vi "Main Window.vi"() -> ()   [LabVIEW 2014]
uses:
  Temp Sensor Folder/Global Stop TempSensor.vi
  StopForLog.vi
panel:
  in  "בחירה חופשית":bool caption="Blank Button"
  in  "ממסר השהייה למפוח מפנה גזים 0410-26308":bool caption="Blank Button"
  in  "ממסר דימום מנוע 0410-26294":bool caption="Blank Button"
  in  "0410-24534 15A ממסר":bool caption="Blank Button"
  in  "0410-19646 10Ax4 ממסר":bool caption="Blank Button"
  in  "תיבת נתיכים סימן 4 0414-83040":bool caption="Blank Button"
  in  "תיבת מפעיל ריצוף 1469-98836":bool caption="Blank Button"
  in  "תיבת הזנה כיס צריח 0410-23813":bool caption="Blank Button"
  in  "Help Button":bool
  in  "Stop Button":bool
  out "error IO":errorcluster
  in  "error":errorcluster
  # "צב\"ד לממסרים ונתיכים"
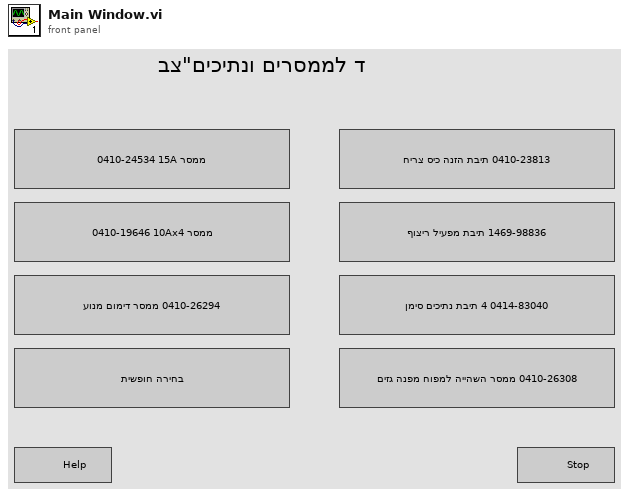
[diagram p1: front panel]
types:
  T1 = enum32{"Invalid", "Standard", "Closed", "Hidden", "Minimized", "Maximized"}
  T2 = enum16{"open", "replace", "create", "open or create", "replace or create", "replace or create with confirmation"}
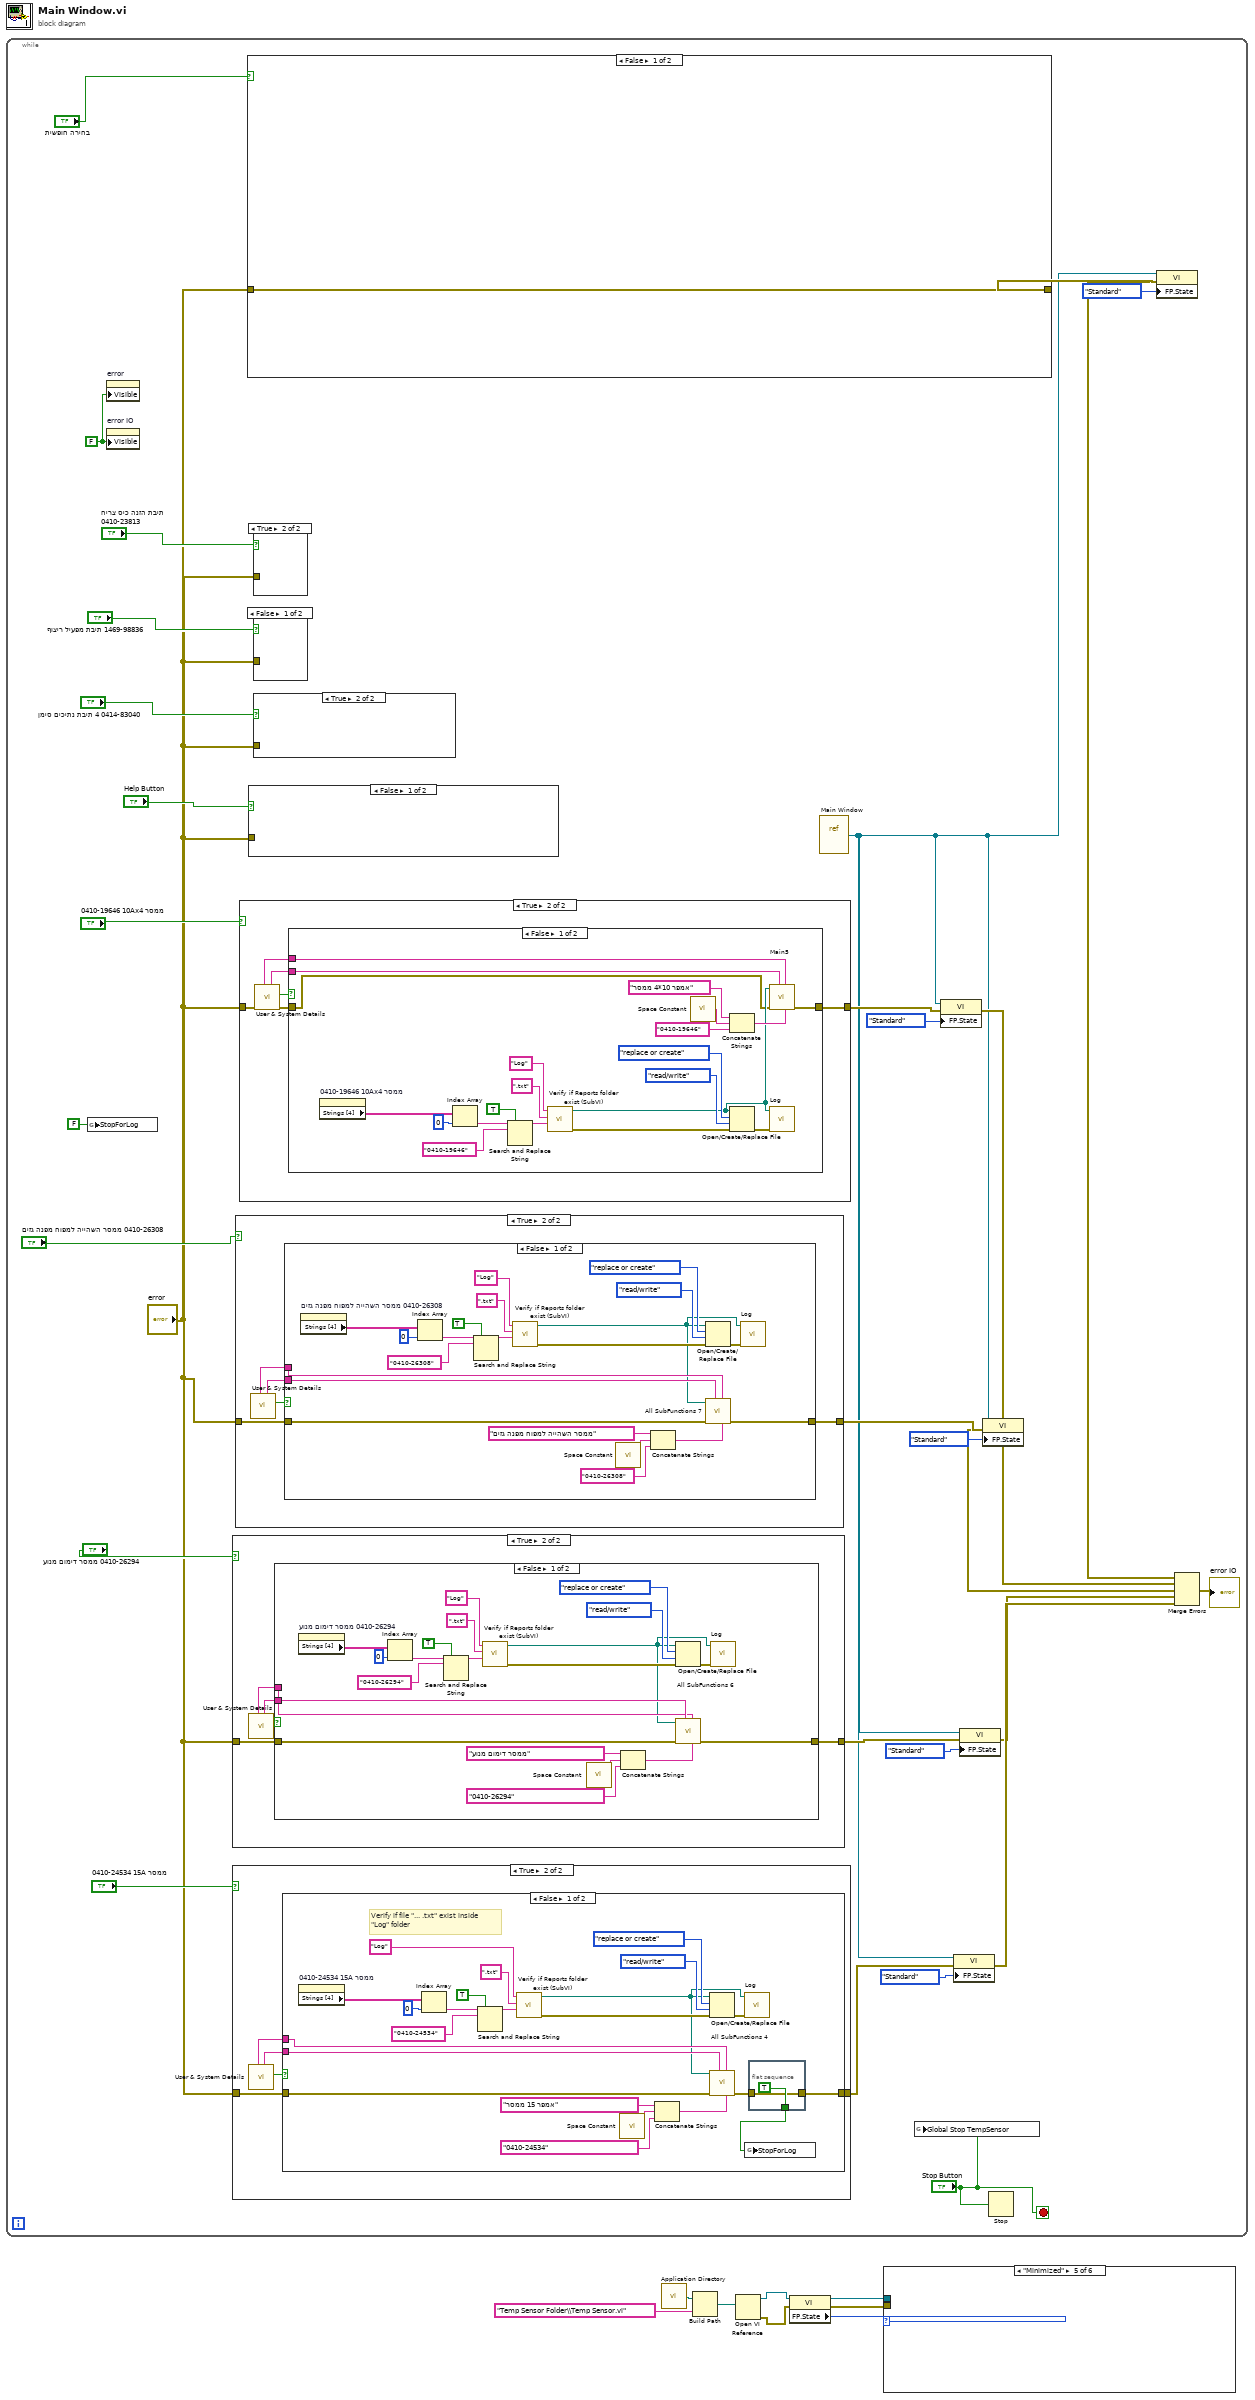
[diagram p0: block diagram]
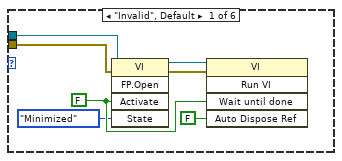
[diagram p2: hidden frame]
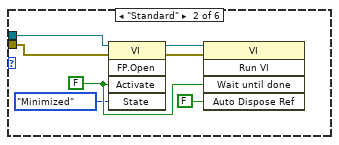
[diagram p3: hidden frame]
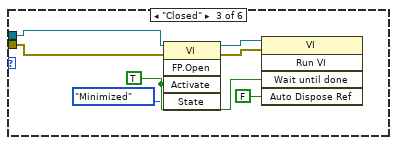
[diagram p4: hidden frame]
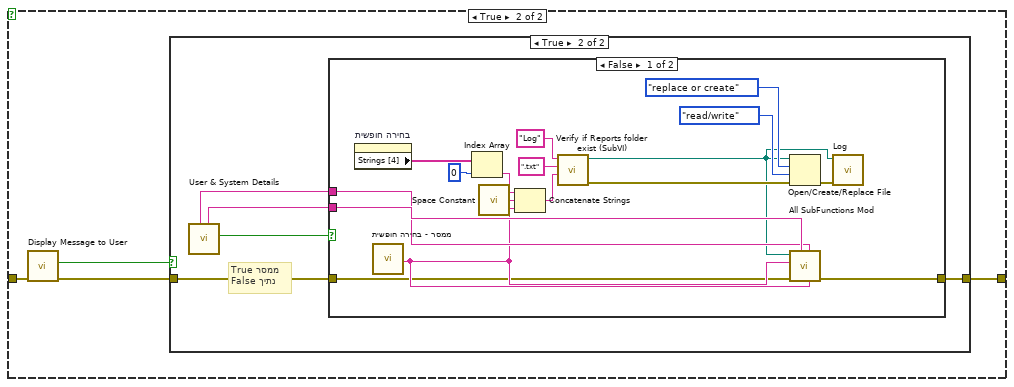
[diagram p7: hidden frame]
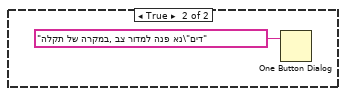
[diagram p10: hidden frame]
diagram:
  n1 = while {
    stop <- "Stop Button" stop-if-true
    w30 = FALSE ("Visible")
    n2 = global write "StopForLog.vi" "StopForLog"(FALSE ("StopForLog")) -> ()
    n3 = property on="error" class="Clust (strict)"("Visible"=w30) -> ()  [unwired: 2 in, 2 out]
    n4 = property on="error IO" class="Clust (strict)"("Visible"=w30) -> ()  [unwired: 2 in, 2 out]
    n5 = case shown="True" "ממסר דימום מנוע 0410-26294" {
      tunnel: "error" -> [w158 w163]
      tunnel: [w158 w162] -> w25
      frame False {
      }
      frame True {
        n6 = call "User & System Details.vi"() -> ("Boolean"=w161:bool, "User Name 2"=w160:string, "מספר סידורי 2"=w159:string)  [unwired: 8 in, 1 out]
        n7 = case shown="False" w161 {
          tunnel: w163 -> [w165 w185]
          tunnel: [w167 w185] -> w162
          tunnel: w160 -> [w169 _]
          tunnel: w159 -> [w168 _]
          frame False {
            n8 = property on="ממסר דימום מנוע 0410-26294" class="Bool"() -> ("Strings [4]"=w176:string[])  [unwired: 2 in, 2 out]
            n9 = Index Array(array=w176, index=0) -> (element=w181:string)
            n10 = Search and Replace String(replace all?=TRUE ("replace all? (F)"), input string=w181, search string="0410-26294") -> (result string=w179:string)  [unwired: 5 in, 3 out]
            n11 = call "Verify if Reports folder exist (SubVI).vi"("שם הממסר"=w179, "File Type"=".txt", "Folder Name"="Log" ("string")) -> ("error out"=w173:errorcluster, "Path"=w164:path)  [unwired: 7 in]
            n12 = call <vilib>:"Space Constant.vi"() -> ("String"=w184:string)
            n13 = Concatenate Strings("ממסר דימום מנוע", w184, "0410-26294") -> (w170:string)
            n14 = Open/Create/Replace File(file path (use dialog)=w164, error in=w173, operation (0:open)=T2."replace or create", access (0:read/write)=enum16{"read/write", "read-only", "write-only"}."read/write") -> (error out=w166:errorcluster)  [unwired: 2 in, 2 out]
            n15 = call "All SubFunctions 6.vi"("מק\"ט המכלל"=w170, "מספר סידורי"=w168, "מפעיל"=w169, "error"=w165, "Path for Log"=w164) -> ("error IO"=w167:errorcluster)  [unwired: 6 in]
            n16 = call "Log.vi"("error in"=w166, "File Path Control"=w164) -> ()  [unwired: 8 in, 2 out]
          }
          frame True {
          }
        }
      }
    }
    n17 = case shown="True" "0410-24534 15A ממסר" {
      tunnel: "error" -> [w69 w70]
      tunnel: [w69 w74] -> w28
      frame False {
      }
      frame True {
        n18 = call "User & System Details.vi"() -> ("Boolean"=w73:bool, "User Name 2"=w72:string, "מספר סידורי 2"=w71:string)  [unwired: 8 in, 1 out]
        n19 = case shown="False" w73 {
          tunnel: [w76 w100] -> w74
          tunnel: w72 -> [w82 _]
          tunnel: w71 -> [w81 _]
          tunnel: w70 -> [w80 w100]
          frame False {
            # "Verify if file \"... .txt\" exist inside\n\"Log\" folder"
            n20 = property on="0410-24534 15A ממסר" class="Bool"() -> ("Strings [4]"=w92:string[])  [unwired: 2 in, 2 out]
            n21 = Index Array(array=w92, index=0) -> (element=w87:string)
            n22 = Search and Replace String(replace all?=TRUE ("replace all? (F)"), input string=w87, search string="0410-24534") -> (result string=w89:string)  [unwired: 5 in, 3 out]
            n23 = call "Verify if Reports folder exist (SubVI).vi"("שם הממסר"=w89, "File Type"=".txt", "Folder Name"="Log" ("string")) -> ("error out"=w95:errorcluster, "Path"=w78:path)  [unwired: 7 in]
            n24 = call <vilib>:"Space Constant.vi"() -> ("String"=w83:string)
            n25 = Concatenate Strings("ממסר 15 אמפר", w83, "0410-24534") -> (w85:string)
            n26 = Open/Create/Replace File(file path (use dialog)=w78, error in=w95, operation (0:open)=T2."replace or create", access (0:read/write)=enum16{"read/write", "read-only", "write-only"}."read/write") -> (error out=w79:errorcluster)  [unwired: 2 in, 2 out]
            n27 = call "All SubFunctions 4.vi"("מק\"ט המכלל"=w85, "מספר סידורי"=w81, "מפעיל"=w82, "error"=w80, "Path for Log"=w78) -> ("error IO"=w77:errorcluster)  [unwired: 6 in]
            n28 = call "Log.vi"("error in"=w79, "File Path Control"=w78) -> ()  [unwired: 8 in, 2 out]
            n29 = global write "StopForLog.vi" "StopForLog"(w75) -> ()
            n30 = flat-sequence {
              tunnel: w77 -> [w98]
              tunnel: [TRUE] -> w75
              tunnel: [w98] -> w76
              frame #0 {
              }
            }
          }
          frame True {
          }
        }
      }
    }
    n31 = case shown="True" "ממסר השהייה למפוח מפנה גזים 0410-26308" {
      tunnel: "error" -> [w130 w135]
      tunnel: [w130 w134] -> w21
      frame False {
      }
      frame True {
        n32 = call "User & System Details.vi"() -> ("Boolean"=w133:bool, "User Name 2"=w132:string, "מספר סידורי 2"=w131:string)  [unwired: 8 in, 1 out]
        n33 = case shown="False" w133 {
          tunnel: w135 -> [w136 w157]
          tunnel: [w139 w157] -> w134
          tunnel: w132 -> [w141 _]
          tunnel: w131 -> [w140 _]
          frame False {
            n34 = property on="ממסר השהייה למפוח מפנה גזים 0410-26308" class="Bool"() -> ("Strings [4]"=w150:string[])  [unwired: 2 in, 2 out]
            n35 = Index Array(array=w150, index=0) -> (element=w145:string)
            n36 = Search and Replace String(replace all?=TRUE ("replace all? (F)"), input string=w145, search string="0410-26308") -> (result string=w147:string)  [unwired: 5 in, 3 out]
            n37 = call "Verify if Reports folder exist (SubVI).vi"("שם הממסר"=w147, "File Type"=".txt", "Folder Name"="Log" ("string")) -> ("error out"=w153:errorcluster, "Path"=w137:path)  [unwired: 7 in]
            n38 = call <vilib>:"Space Constant.vi"() -> ("String"=w144:string)
            n39 = Concatenate Strings("ממסר השהייה למפוח מפנה גזים", w144, "0410-26308") -> (w156:string)
            n40 = Open/Create/Replace File(file path (use dialog)=w137, error in=w153, operation (0:open)=T2."replace or create", access (0:read/write)=enum16{"read/write", "read-only", "write-only"}."read/write") -> (error out=w138:errorcluster)  [unwired: 2 in, 2 out]
            n41 = call "All SubFunctions 7.vi"("מק\"ט המכלל"=w156, "מספר סידורי"=w140, "מפעיל"=w141, "error"=w136, "Path for Log"=w137) -> ("error IO"=w139:errorcluster)  [unwired: 6 in]
            n42 = call "Log.vi"("error in"=w138, "File Path Control"=w137) -> ()  [unwired: 8 in, 2 out]
          }
          frame True {
          }
        }
      }
    }
    n43 = case shown="True" "0410-19646 10Ax4 ממסר" {
      tunnel: "error" -> [w101 w102]
      tunnel: [w101 w107] -> w18
      frame False {
      }
      frame True {
        n44 = call "User & System Details.vi"("error in (no error)"=w102) -> ("error out"=w103:errorcluster, "Boolean"=w106:bool, "User Name 2"=w105:string, "מספר סידורי 2"=w104:string)  [unwired: 7 in]
        n45 = case shown="False" w106 {
          tunnel: [w108 w129] -> w107
          tunnel: w105 -> [w113 _]
          tunnel: w104 -> [w112 _]
          tunnel: w103 -> [w109 w129]
          frame False {
            n46 = property on="0410-19646 10Ax4 ממסר" class="Bool"() -> ("Strings [4]"=w120:string[])  [unwired: 2 in, 2 out]
            n47 = Index Array(array=w120, index=0) -> (element=w125:string)
            n48 = Search and Replace String(replace all?=TRUE ("replace all? (F)"), input string=w125, search string="0410-19646") -> (result string=w123:string)  [unwired: 5 in, 3 out]
            n49 = call "Verify if Reports folder exist (SubVI).vi"("שם הממסר"=w123, "File Type"=".txt", "Folder Name"="Log" ("string")) -> ("error out"=w117:errorcluster, "Path"=w111:path)  [unwired: 7 in]
            n50 = call <vilib>:"Space Constant.vi"() -> ("String"=w126:string)
            n51 = Concatenate Strings("ממסר 4*10 אמפר", w126, "0410-19646") -> (w114:string)
            n52 = Open/Create/Replace File(file path (use dialog)=w111, error in=w117, operation (0:open)=T2."replace or create", access (0:read/write)=enum16{"read/write", "read-only", "write-only"}."read/write") -> (error out=w110:errorcluster)  [unwired: 2 in, 2 out]
            n53 = call "Main5.vi"("מק\"ט המכלל"=w114, "מספר סידורי"=w112, "מפעיל"=w113, "error"=w109, "Path for Log"=w111) -> ("error IO"=w108:errorcluster)  [unwired: 6 in]
            n54 = call "Log.vi"("error in"=w110, "File Path Control"=w111) -> ()  [unwired: 8 in, 2 out]
          }
          frame True {
          }
        }
      }
    }
    n55 = case shown="False" "בחירה חופשית" {
      tunnel: "error" -> [w39 w42]
      tunnel: [w39 w40] -> w13
      frame False {
      }
      frame True {
        n56 = call "Display Message to User"("error in (no error)"=w42) -> ("error out"=w41:errorcluster, "ממסר"=w43:bool)  [unwired: 9 in]
        n57 = case shown="True" w43 {
          tunnel: w41 -> [w44 w47]
          tunnel: [w44 w45] -> w40
          frame False {
          }
          frame True {
            # "True ממסר\nFalse נתיך"
            n58 = call "User & System Details.vi"() -> ("Boolean"=w46:bool, "User Name 2"=w49:string, "מספר סידורי 2"=w48:string)  [unwired: 8 in, 1 out]
            n59 = case shown="False" w46 {
              tunnel: w47 -> [w50 w67]
              tunnel: [w51 w67] -> w45
              tunnel: w49 -> [w61 _]
              tunnel: w48 -> [w60 _]
              frame False {
                n60 = property on="בחירה חופשית" class="Bool"() -> ("Strings [4]"=w59:string[])  [unwired: 2 in, 2 out]
                n61 = call "בחירה חופשית - ממסר"() -> ("שם הממסר"=w54:string)  [unwired: 17 in, 2 out]
                n62 = Index Array(array=w59, index=0) -> (element=w57:string)
                n63 = call <vilib>:"Space Constant.vi"() -> ("String"=w56:string)
                n64 = Concatenate Strings(w57, w56, w54) -> (w55:string)
                n65 = call "Verify if Reports folder exist (SubVI).vi"("שם הממסר"=w55, "File Type"=".txt", "Folder Name"="Log" ("string")) -> ("error out"=w64:errorcluster, "Path"=w52:path)  [unwired: 7 in]
                n66 = Open/Create/Replace File(file path (use dialog)=w52, error in=w64, operation (0:open)=T2."replace or create", access (0:read/write)=enum16{"read/write", "read-only", "write-only"}."read/write") -> (error out=w53:errorcluster)  [unwired: 2 in, 2 out]
                n67 = call "All SubFunctions Mod.vi"("מק\"ט המכלל"=w54, "מספר סידורי"=w60, "מפעיל"=w61, "error"=w50, "שם הממסר"=w54, "Path for Log"=w52) -> ("error IO"=w51:errorcluster)  [unwired: 5 in]
                n68 = call "Log.vi"("error in"=w53, "File Path Control"=w52) -> ()  [unwired: 8 in, 2 out]
              }
              frame True {
              }
            }
          }
        }
      }
    }
    n69 = case shown="False" "Help Button" {
      tunnel: "error" -> [_ _]
      frame False {
      }
      frame True {
        n70 = One Button Dialog(message="במקרה של תקלה, נא פנה למדור צב\"דים") -> ()  [unwired: 1 in, 1 out]
      }
    }
    n71 = case shown="True" "תיבת הזנה כיס צריח 0410-23813" {
      tunnel: "error" -> [_ _]
      frame False {
      }
      frame True {
      }
    }
    n72 = case shown="False" "תיבת מפעיל ריצוף 1469-98836" {
      tunnel: "error" -> [_ _]
      frame False {
      }
      frame True {
      }
    }
    n73 = case shown="True" "תיבת נתיכים סימן 4 0414-83040" {
      tunnel: "error" -> [_ _]
      frame False {
      }
      frame True {
      }
    }
    n74 = vi-ref "Main Window.vi"() -> (w9:refnum<vi>)
    n75 = global write "Global Stop TempSensor.vi" "Global Stop TempSensor"("Stop Button") -> ()
    n76 = property class="VI"(reference=w9, error in=w18, "FP.State"=T1."Standard" ("Front Panel Window:State")) -> (error out=w17:errorcluster)  [unwired: 1 out]
    n77 = property class="VI"(reference=w9, error in=w28, "FP.State"=T1."Standard" ("Front Panel Window:State")) -> (error out=w26:errorcluster)  [unwired: 1 out]
    n78 = property class="VI"(reference=w9, error in=w25, "FP.State"=T1."Standard" ("Front Panel Window:State")) -> (error out=w24:errorcluster)  [unwired: 1 out]
    n79 = property class="VI"(reference=w9, error in=w21, "FP.State"=T1."Standard" ("Front Panel Window:State")) -> (error out=w20:errorcluster)  [unwired: 1 out]
    n80 = Stop(stop? (T)="Stop Button") -> ()
    n81 = property class="VI"(reference=w9, error in=w13, "FP.State"=T1."Standard" ("Front Panel Window:State")) -> (error out=w12:errorcluster)  [unwired: 1 out]
    n82 = Merge Errors(w12, w17, w20, w24, w26) -> (→"error IO":errorcluster)
  }
  n83 = call <vilib>:"Application Directory.vi"() -> ("Application Directory"=w8:path)
  n84 = Build Path(base path=w8, name or relative path="Temp Sensor Folder\\Temp Sensor.vi") -> (appended path=w6:path)
  n85 = Open VI Reference(vi path=w6) -> (vi reference=w5:refnum<vi>, error out=w4:errorcluster)  [unwired: 5 in]
  n86 = property class="VI"(reference=w5, error in=w4) -> (reference out=w1:refnum<vi>, error out=w2:errorcluster, "FP.State"=w3:T1)
  n87 = case shown="\"Minimized\"" w3 {
    tunnel: w2 -> [w187 w194 w201 _ _ _]
    tunnel: w1 -> [w186 w193 w200 _ _ _]
    frame "Invalid", Default {
      w192 = FALSE ("Wait Until Done")
      n88 = invoke class="VI" method="FP.Open"(reference=w186, error in=w187, "Activate"=w192, "State"=T1."Minimized") -> (reference out=w189:refnum<vi>, error out=w190:errorcluster)  [unwired: 1 in, 3 out]
      n89 = invoke class="VI" method="Run VI"(reference=w189, error in=w190, "Wait until done"=w192, "Auto Dispose Ref"=FALSE ("Auto Dispose Reference")) -> ()  [unwired: 1 in, 5 out]
    }
    frame "Standard" {
      w199 = FALSE ("Wait Until Done")
      n90 = invoke class="VI" method="FP.Open"(reference=w193, error in=w194, "Activate"=w199, "State"=T1."Minimized") -> (reference out=w196:refnum<vi>, error out=w197:errorcluster)  [unwired: 1 in, 3 out]
      n91 = invoke class="VI" method="Run VI"(reference=w196, error in=w197, "Wait until done"=w199, "Auto Dispose Ref"=FALSE ("Auto Dispose Reference")) -> ()  [unwired: 1 in, 5 out]
    }
    frame "Closed" {
      w206 = TRUE ("Wait Until Done")
      n92 = invoke class="VI" method="FP.Open"(reference=w200, error in=w201, "Activate"=w206, "State"=T1."Minimized") -> (reference out=w203:refnum<vi>, error out=w204:errorcluster)  [unwired: 1 in, 3 out]
      n93 = invoke class="VI" method="Run VI"(reference=w203, error in=w204, "Wait until done"=w206, "Auto Dispose Ref"=FALSE ("Auto Dispose Reference")) -> ()  [unwired: 1 in, 5 out]
    }
    frame "Hidden" {
    }
    frame "Minimized" {
    }
    frame "Maximized" {
    }
  }
